vi "S2C_Access_DBVersion.vi"(7 "Action":enum16{"Get", "Set"}(ring), 8 "Error In":errorcluster) -> (0 "Error Out":errorcluster, 3 "Data Out":string)   [LabVIEW 2015]
uses:
  S2C_Access_Globals.vi
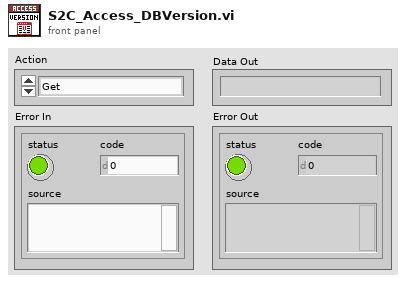
[diagram p1: front panel]
types:
  T1 = cluster{"Version":string, "LastUpdate":string, "ModifiedBy":string}
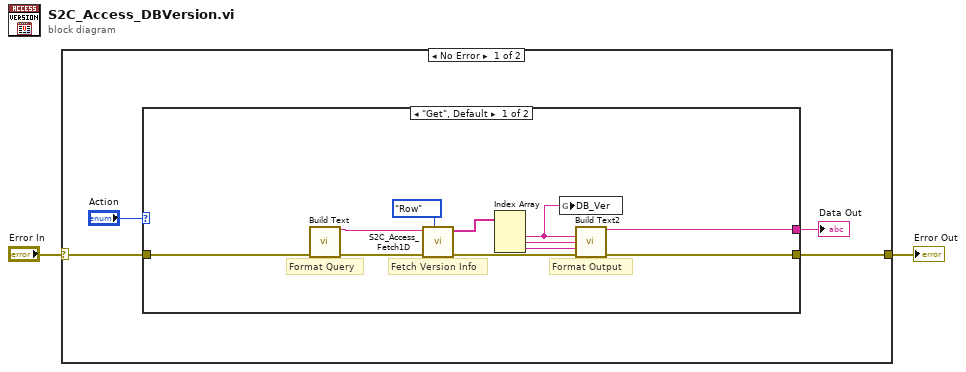
[diagram p0: block diagram]
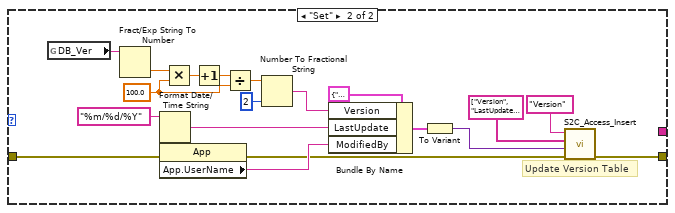
[diagram p2: hidden frame]
diagram:
  n1 = case shown="No Error" "Error In" {
    selector: "Error In" -> [w6 w37]
    tunnel: [w5 w37] -> w1
    frame No Error {
      n2 = case shown="\"Get\", Default" "Action" {
        tunnel: w6 -> [w17 w20]
        tunnel: [w10 w33] -> w5
        tunnel: [w9 _] -> w3
        frame "Get", Default {
          # "Format Output"
          # "Fetch Version Info"
          # "Format Query"
          n3 = call "Build Text"("error in (no error)"=w17) -> ("Result"=w15:string, "error out"=w16:errorcluster)  [unwired: 13 in]
          n4 = call "S2C_Access_Fetch1D.vi"("Selection"=enum16{"Row", "Col"}."Row", "Error In"=w16, "Query"=w15) -> ("Error Out"=w13:errorcluster, "Data"=w14:string[])  [unwired: 7 in]
          n5 = Index Array(array=w14) -> (element #1=w7:string, element #2=w11:string, element #3=w12:string)  [unwired: 3 in]
          n6 = global write "S2C_Access_Globals.vi" "DB_Ver"(w7) -> ()
          n7 = call "Build Text2"("Ver"=w7, "Update"=w11, "ModBy"=w12, "error in (no error)"=w13) -> ("Result"=w9:string, "error out"=w10:errorcluster)  [unwired: 10 in]
        }
        frame "Set" {
          w25 = 100.0 ("y")
          # "Update Version Table"
          n8 = global read "S2C_Access_Globals.vi" "DB_Ver"() -> (w28:string)
          n9 = Fract/Exp String To Number(string=w28) -> (number=w22:dbl)  [unwired: 3 in, 1 out]
          n10 = Format Date/Time String(time format string (%c)="%m/%d/%Y") -> (date/time string=w30:string)  [unwired: 2 in]
          n11 = property class="App"(error in=w20) -> (error out=w19:errorcluster, "App.UserName"=w32:string)  [unwired: 1 in, 1 out]
          n12 = Multiply(x=w22, y=w25) -> (x*y=w23:dbl)
          n13 = Increment(x=w23) -> (x+1=w24:dbl)
          n14 = Divide(x=w24, y=w25) -> (x/y=w26:dbl)
          n15 = Number To Fractional String(number=w26, precision (6)=i16 2) -> (F-format string=w31:string)  [unwired: 2 in]
          n16 = Bundle By Name(cluster=T1 {"Version"="", "LastUpdate"="", "ModifiedBy"=""}, "Version"=w31, "LastUpdate"=w30, "ModifiedBy"=w32) -> (w18:T1)
          n17 = To Variant(anything=w18) -> (Variant=w34:variant)
          n18 = call "S2C_Access_Insert.vi"("Error In"=w19, "Data"=w34, "Columns"=string[] ["Version", "LastUpdate", "ModifiedBy"], "Table"="Version") -> ("Error Out"=w33:errorcluster)  [unwired: 7 in]
        }
      }
      "Data Out" <- w3
    }
    frame Error {
    }
  }
  "Error Out" <- w1
